vi "UI - Initiate Connection.vi"(8 "error in (no error)":errorcluster, 10 "Controller Address":string, 11 "Message Queue":refnum<queue>) -> (0 "error out":errorcluster, 1 "Connected?":bool)   [LabVIEW 2017]
uses:
  Message Queue/Message Cluster.ctl
  controls/FPGA State.ctl
  controls/CPU Loads.ctl
  <vilib>/vision/Image Controls.llb/IMAQ Image.ctl
  Globals/Global - Configuration Options.vi
  Globals/Global - UI Stream and Variable Connections.vi
  Message Queue/Message Queue.lvlib
panel:
  out "error out 4":errorcluster
  out "error out 3":errorcluster
  out "error out 2":errorcluster
  out "tag acc":refnum<k21>
  out "Tag acc":refnum<k21>
  out "Variable Name Control/Indicator 2":refnum<k21>
  out "Variable Name Control/Indicator":refnum<k21>
  out "resulting string 2":string
  out "reader name":string="UI Reader"
  out "writer name":string="UI Writer"
  out "resulting string":string
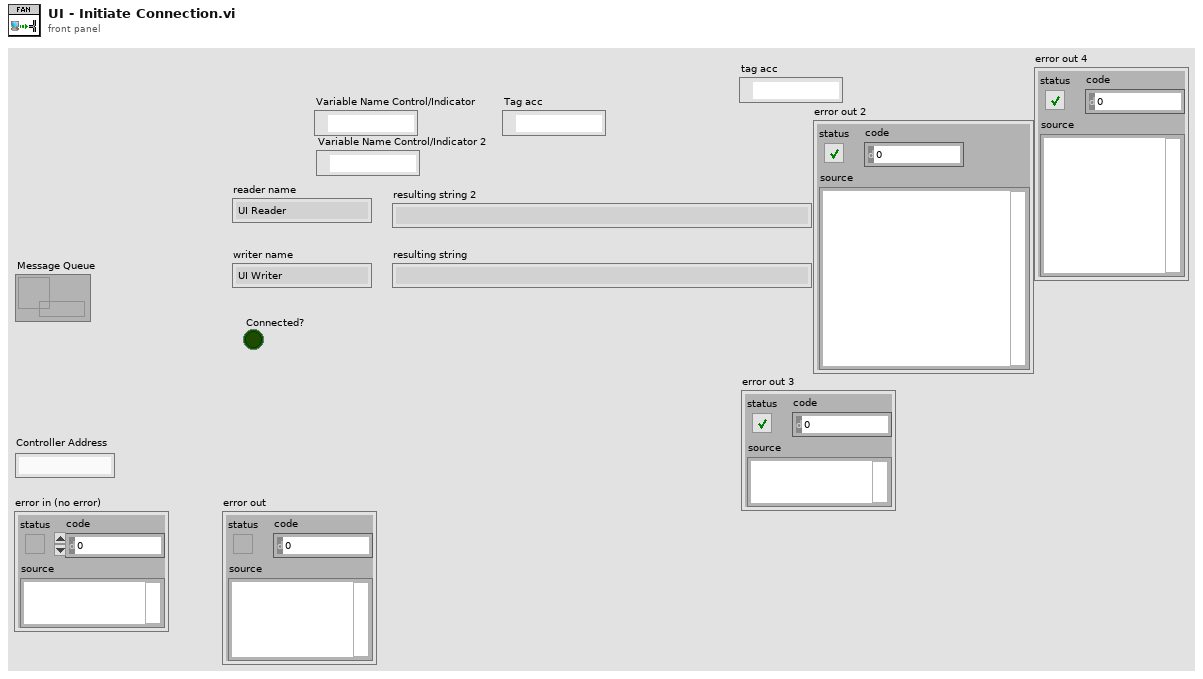
[diagram p1: front panel]
types:
  T1 = typedef "IMAQ Image.ctl" = refnum<image>
  T2 = typedef "CPU Loads.ctl" = cluster{"Total (%)":dbl, "Time Critical (%)":dbl, "Timed Structures (%)":dbl, "High (%)":dbl, "Above Normal (%)":dbl, "Normal (%)":dbl, "Background (%)":dbl, "Idle (%)":dbl, "ISR (%)":dbl}[]
  T3 = typedef "FPGA State.ctl" = enum16{"Safe State", "Control (PID)"}
  T4 = typedef "Message Queue.lvlib/Message Cluster.ctl" = cluster{"Message":string, "Message Data":variant}
  T5 = cluster{"Actual PID Loop Period":refnum<k21>, "DMA FIFO Overflow?":refnum<k21>, "CPU Usage":refnum<k21>, "Free or Contiguous Memory":refnum<k21>, "Current FPGA State":refnum<k21>, "Acceleration (grms)":refnum<k21>, "Acceleration Waveform":refnum<k21>, "Chatter":refnum<k21>, "tag acc":refnum<k21>, "tag video":refnum<k21>, "images":refnum<k21>}
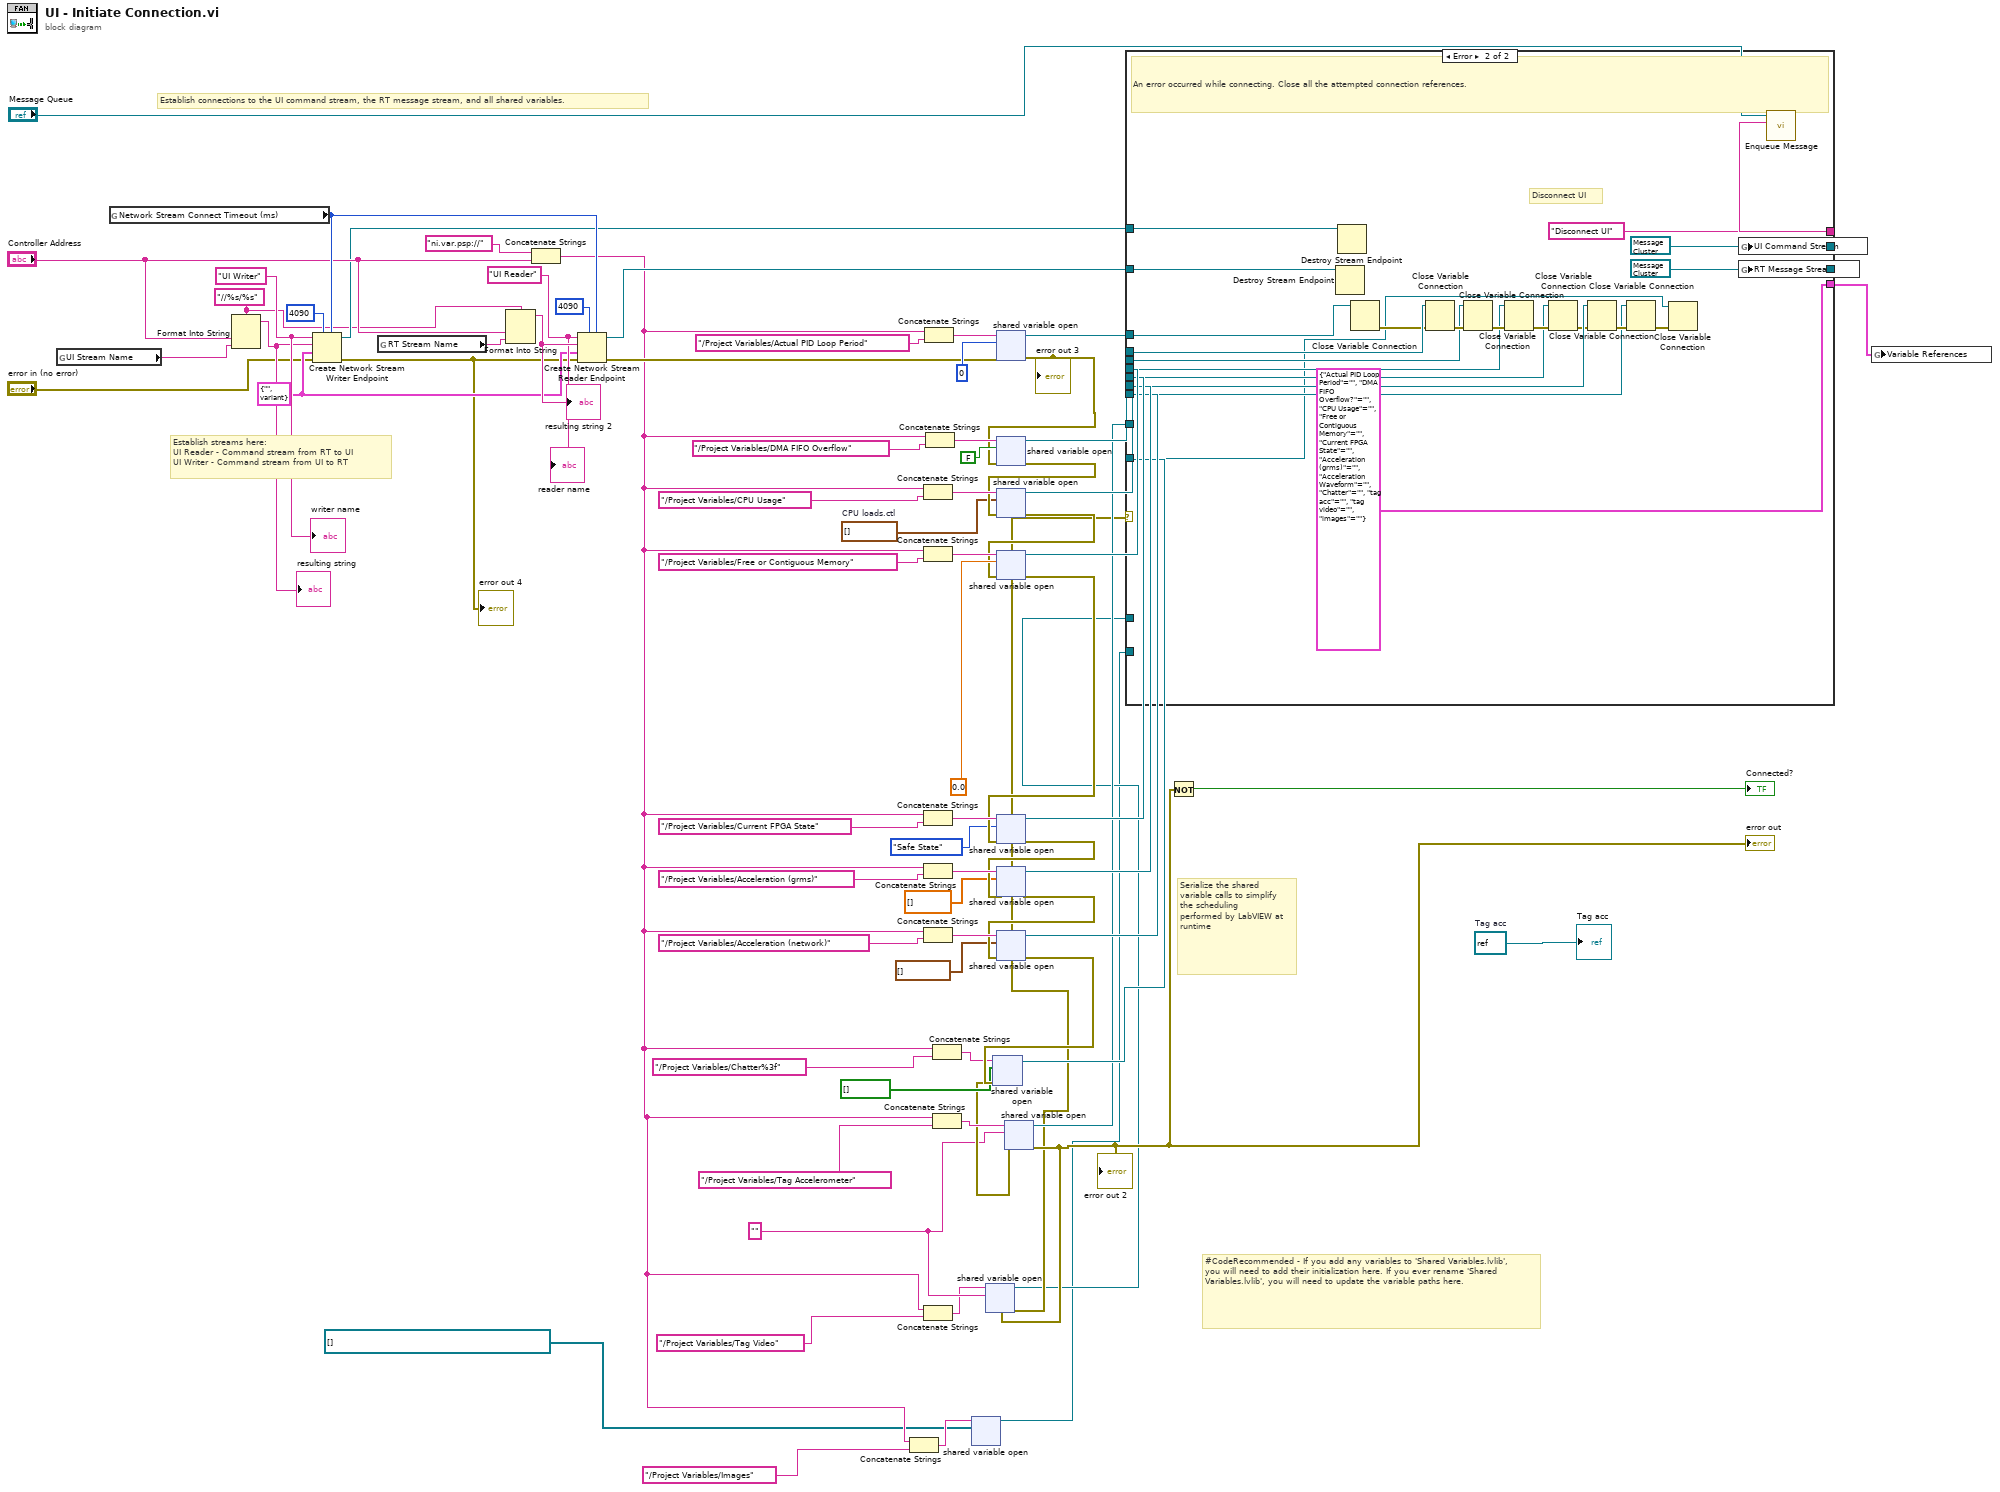
[diagram p0: block diagram]
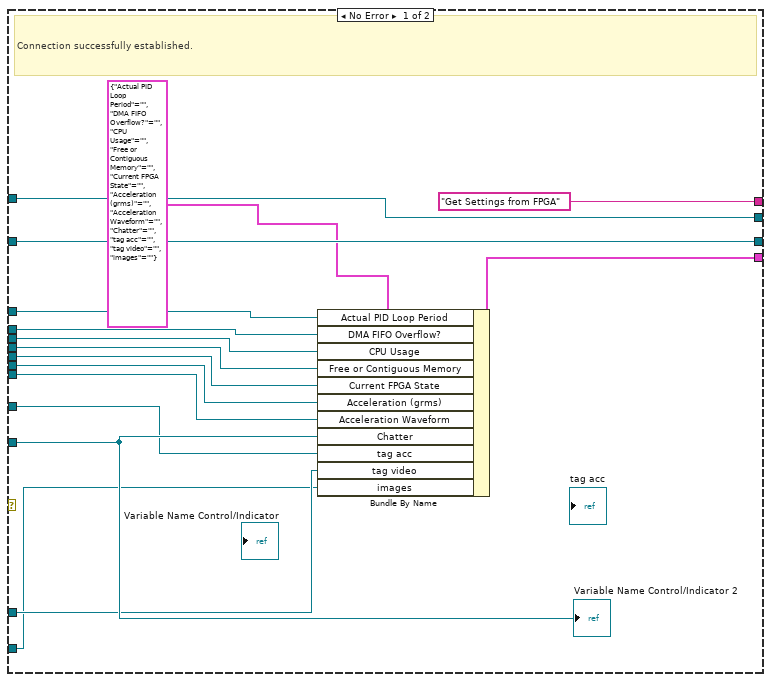
[diagram p2: hidden frame]
diagram:
  w12 = "" ("string")
  w14 = refnum<k21> refnum  # Tag acc
  w29 = T2 []  # CPU loads.ctl
  w74 = T4 {"Message"="", "Message Data"=variant} ("Message Cluster")
  w75 = "UI Reader" ("reader name")
  w78 = "UI Writer" ("writer name")
  w21 = "//%s/%s"
  # "Establish connections to the UI command stream, the RT message stream, and all shared variables."
  # "#CodeRecommended - If you add any variables to 'Shared Variables.lvlib', you will need to add their initialization here. If you ever rename 'Shared Variables.lvlib', you will need to update the variable paths here."
  # "Establish streams here:\nUI Reader - Command stream from RT to UI\nUI Writer - Command stream from UI to RT"
  # "Serialize the shared variable calls to simplify the scheduling performed by LabVIEW at runtime"
  n1 = global read "Global - Configuration Options.vi" "UI Stream Name"() -> (w20:string)
  n2 = global read "Global - Configuration Options.vi" "Network Stream Connect Timeout (ms)"() -> (w73:i32)
  n3 = Format Into String(format string=w21, "Controller Address", w20) -> (resulting string=w77:string)  [unwired: 2 in, 1 out]
  "resulting string" <- w77
  n4 = Create Network Stream Writer Endpoint(5:w73, 7:4090 ("writer buffer size"), 8:"error in (no error)", 9:w74, 10:w77, 11:w78) -> (0:w7:errorcluster, 3:w59:refnum<k21>)  [unwired: 1 in]
  "error out 4" <- w7
  n5 = global read "Global - Configuration Options.vi" "RT Stream Name"() -> (w19:string)
  n6 = Format Into String(format string=w21, "Controller Address", w19) -> (resulting string=w76:string)  [unwired: 2 in, 1 out]
  "resulting string 2" <- w76
  n7 = Concatenate Strings("ni.var.psp://", "Controller Address") -> (w4:string)
  n8 = Create Network Stream Reader Endpoint(5:w73, 7:4090 ("reader buffer size"), 8:w7, 9:w74, 10:w76, 11:w75) -> (0:w52:errorcluster, 3:w58:refnum<k21>)  [unwired: 1 in]
  n9 = Concatenate Strings(w4, "/Project Variables/Images") -> (w6:string)
  n10 = Concatenate Strings(w4, "/Project Variables/CPU Usage") -> (w64:string)
  n11 = Concatenate Strings(w4, "/Project Variables/Free or Contiguous Memory") -> (w48:string)
  n12 = Concatenate Strings(w4, "/Project Variables/Current FPGA State") -> (w45:string)
  n13 = Concatenate Strings(w4, "/Project Variables/Acceleration (grms)") -> (w44:string)
  n14 = Concatenate Strings(w4, "/Project Variables/Acceleration (network)") -> (w41:string)
  n15 = Concatenate Strings(w4, "/Project Variables/Tag Video") -> (w8:string)
  n16 = Concatenate Strings(w4, "/Project Variables/Actual PID Loop Period") -> (w69:string)
  n17 = Concatenate Strings(w4, "/Project Variables/DMA FIFO Overflow") -> (w67:string)
  n18 = Concatenate Strings(w4, "/Project Variables/Chatter%3f") -> (w24:string)
  n19 = Concatenate Strings(w4, "/Project Variables/Tag Accelerometer") -> (w18:string)
  n20 = shared-variable-open(w6, T1[] []) -> (w2:refnum<k21>)  [unwired: 2 in, 1 out]
  n21 = shared-variable-open(w69, w52, u32 0) -> (w62:refnum<k21>, w22:errorcluster)  [unwired: 1 in]
  "error out 3" <- w22
  n22 = shared-variable-open(w67, w22, FALSE ("data type")) -> (w61:refnum<k21>, w63:errorcluster)  [unwired: 1 in]
  n23 = shared-variable-open(w64, w63, w29) -> (w60:refnum<k21>, w40:errorcluster)  [unwired: 1 in]
  n24 = shared-variable-open(w48, w40, 0.0) -> (w35:refnum<k21>, w39:errorcluster)  [unwired: 1 in]
  n25 = shared-variable-open(w45, w39, FPGA_State."Safe State" ("FPGA State")) -> (w34:refnum<k21>, w38:errorcluster)  [unwired: 1 in]
  n26 = shared-variable-open(w44, w38, dbl[] []) -> (w33:refnum<k21>, w37:errorcluster)  [unwired: 1 in]
  n27 = shared-variable-open(w41, w37, waveform(dbl)[] []) -> (w32:refnum<k21>, w26:errorcluster)  [unwired: 1 in]
  n28 = shared-variable-open(w24, w26, bool[] []) -> (w23:refnum<k21>, w15:errorcluster)  [unwired: 1 in]
  n29 = shared-variable-open(w18, w15, w12) -> (w16:refnum<k21>, w11:errorcluster)  [unwired: 1 in]
  "error out" <- w11
  "error out 2" <- w11
  n30 = shared-variable-open(w8, w11, w12) -> (w9:refnum<k21>, w10:errorcluster)  [unwired: 1 in]
  n31 = case shown="Error" w10 {
    tunnel: w62 -> [w95 w113]
    tunnel: w61 -> [w91 w111]
    tunnel: w60 -> [w90 w112]
    tunnel: w59 -> [w92 w115]
    tunnel: w58 -> [w94 w116]
    tunnel: [w94 refnum<k21> refnum] -> w57
    tunnel: [w92 refnum<k21> refnum] -> w56
    tunnel: ["Get Settings from FPGA" "Disconnect UI"] -> w54
    tunnel: w35 -> [w89 w105]
    tunnel: w34 -> [w88 w104]
    tunnel: w33 -> [w87 w103]
    tunnel: w32 -> [w86 w100]
    tunnel: w23 -> [w85 w97]
    tunnel: w16 -> [w82 _]
    tunnel: [w83 T5 {"Actual PID Loop Period"="", "DMA FIFO Overflow?"="", "CPU Usage"="", "Free or Contiguous Memory"="", "Current FPGA State"="", "Acceleration (grms)"="", "Acceleration Waveform"="", "Chatter"="", "tag acc"="", "tag video"="", "images"=""} ("Variable References")] -> w1
    tunnel: w9 -> [w81 _]
    tunnel: w2 -> [w80 _]
    frame No Error {
      # "Connection successfully established."
      n32 = Bundle By Name(cluster=T5 {"Actual PID Loop Period"="", "DMA FIFO Overflow?"="", "CPU Usage"="", "Free or Contiguous Memory"="", "Current FPGA State"="", "Acceleration (grms)"="", "Acceleration Waveform"="", "Chatter"="", "tag acc"="", "tag video"="", "images"=""} ("Variable References"), "Actual PID Loop Period"=w95, "DMA FIFO Overflow?"=w91, "CPU Usage"=w90, "Free or Contiguous Memory"=w89, "Current FPGA State"=w88, "Acceleration (grms)"=w87, "Acceleration Waveform"=w86, "Chatter"=w85, "tag acc"=w82, "tag video"=w81, "images"=w80) -> (w83:T5)
      "Variable Name Control/Indicator 2" <- w85
    }
    frame Error {
      # "Disconnect UI"
      # "An error occurred while connecting. Close all the attempted connection references."
      n33 = Destroy Stream Endpoint(11:w116) -> ()  [unwired: 1 in, 1 out]
      n34 = Destroy Stream Endpoint(11:w115) -> ()  [unwired: 1 in, 1 out]
      n35 = Close Variable Connection(11:w113) -> (0:w99:errorcluster)  [unwired: 1 in]
      n36 = Close Variable Connection(8:w99, 11:w111) -> (0:w114:errorcluster)
      n37 = Close Variable Connection(8:w114, 11:w112) -> (0:w107:errorcluster)
      n38 = Close Variable Connection(8:w107, 11:w105) -> (0:w106:errorcluster)
      n39 = Close Variable Connection(8:w106, 11:w104) -> (0:w102:errorcluster)
      n40 = Close Variable Connection(8:w102, 11:w103) -> (0:w101:errorcluster)
      n41 = Close Variable Connection(8:w101, 11:w100) -> (0:w98:errorcluster)
      n42 = Close Variable Connection(8:w98, 11:w97) -> ()  [unwired: 1 out]
    }
  }
  n43 = Not(x=w11) -> (.not. x?=→"Connected?":bool)
  n44 = global write "Global - UI Stream and Variable Connections.vi" "UI Command Stream"(w56) -> ()
  n45 = global write "Global - UI Stream and Variable Connections.vi" "RT Message Stream"(w57) -> ()
  n46 = call "Enqueue Message.vi"("Message"=w54, "Message Queue"="Message Queue") -> ()  [unwired: 8 in, 2 out]
  n47 = global write "Global - UI Stream and Variable Connections.vi" "Variable References"(w1) -> ()
  "writer name" <- w78
  "reader name" <- w75
  "Tag acc" <- w14
